vi "NT Read Value.vi"   [LabVIEW 2025]
doc: "A polyVI that will return the data of the named entry. Use the poly selector to choose the type to read."
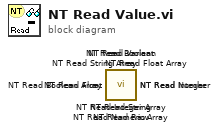
[diagram p0: block diagram]
diagram:
  n1 = call <vilib>:"NT Read Integer Array.vi"() -> ()  [unwired: 9 in, 3 out]
  n2 = call <vilib>:"NT Read Float Array.vi"() -> ()  [unwired: 9 in, 3 out]
  n3 = call <vilib>:"NT Read Float.vi"() -> ()  [unwired: 9 in, 3 out]
  n4 = call <vilib>:"NT Read Integer.vi"() -> ()  [unwired: 9 in, 3 out]
  n5 = call <vilib>:"NT Read Raw.vi"() -> ()  [unwired: 10 in, 2 out]
  n6 = call <vilib>:"NT Read Variant.vi"() -> ()  [unwired: 10 in, 2 out]
  n7 = call <vilib>:"NT Read String Array.vi"() -> ()  [unwired: 9 in, 3 out]
  n8 = call <vilib>:"NT Read Numeric Array.vi"() -> ()  [unwired: 9 in, 3 out]
  n9 = call <vilib>:"NT Read Boolean Array.vi"() -> ()  [unwired: 9 in, 3 out]
  n10 = call <vilib>:"NT Read String.vi"() -> ()  [unwired: 9 in, 3 out]
  n11 = call <vilib>:"NT Read Number.vi"() -> ()  [unwired: 9 in, 3 out]
  n12 = call <vilib>:"NT Read Boolean.vi"() -> ()  [unwired: 9 in, 3 out]
